vi "MoveAI.vi"(7 "ReturnHome(F)":bool, 8 "error in (no error)":errorcluster, 10 "Ball":refnum<class "PongBall.lvclass">, 11 "BouncePanel in":refnum<class "BouncePanel.lvclass">) -> (0 "error out":errorcluster, 3 "BouncePanel out":refnum<class "BouncePanel.lvclass">)   [LabVIEW 2019, in "RT_Game.lvlib" / "BouncePanel.lvclass"]
uses:
  BouncePanel.lvclass
  C:/Users/FreshBob/Dropbox/VIs/myRIO_GameConsole/RT/RT_Game/PongPanel/PongPanel.lvclass
  C:/Users/FreshBob/Dropbox/VIs/myRIO_GameConsole/RT/RT_Game/GameObject/GameObject.lvclass
  PongBall/PongBall.lvclass
  PongPanel/PongPanel.lvclass/PongPanel.ctl
  GameObject/GameObject.lvclass/GameObject.ctl
  PongPanel/Read StartPos.vi
  GameObject/Read Velocity.vi
  PongPanel/PongPanel.lvclass
  GameObject/GameObject.lvclass
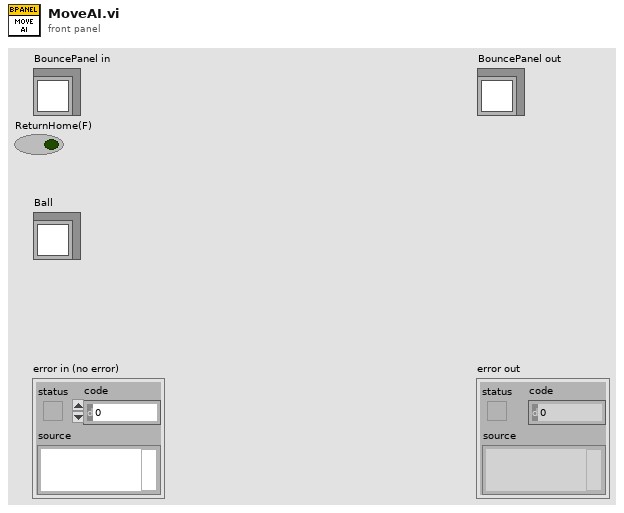
[diagram p1: front panel]
types:
  T1 = typedef "RT_Game.lvlib/Engine.lvclass/Coordinate.ctl" = cluster{"x":dbl, "y":dbl}
  T2 = typedef "Velocity.ctl" = cluster{"x":dbl, "y":dbl}
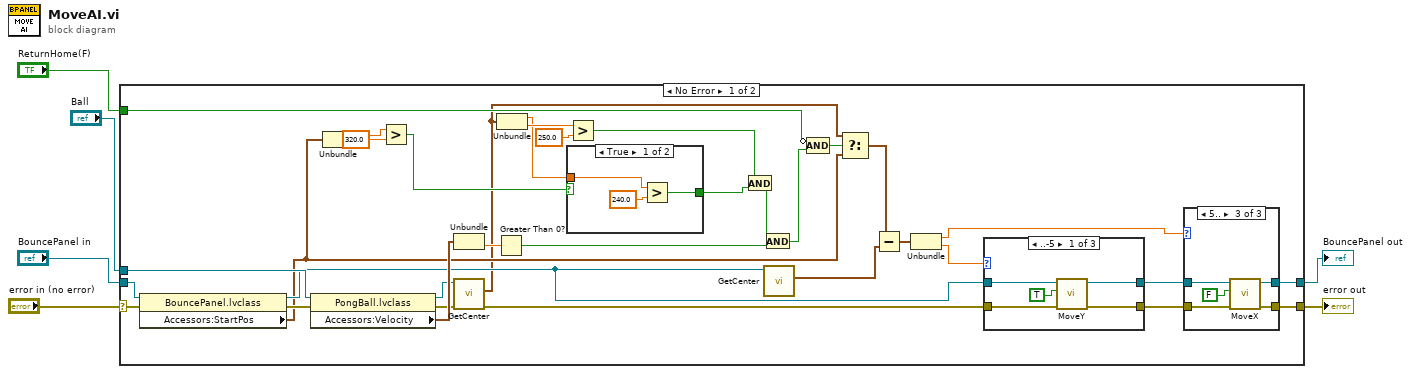
[diagram p0: block diagram]
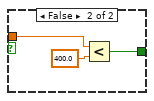
[diagram p2: hidden frame]
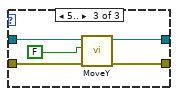
[diagram p4: hidden frame]
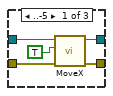
[diagram p5: hidden frame]
diagram:
  n1 = case shown="No Error" "error in (no error)" {
    selector: "error in (no error)" -> [w27 w72]
    tunnel: [w40 w72] -> w3
    tunnel: [w39 w71] -> w4
    tunnel: "BouncePanel in" -> [w22 w71]
    tunnel: "Ball" -> [w38 _]
    tunnel: "ReturnHome(F)" -> [w21 _]
    frame No Error {
      n2 = property class="BouncePanel.lvclass"(reference=w22, error in=w27) -> (reference out=w20:refnum<class "BouncePanel.lvclass">, error out=w23:errorcluster, "Accessors:StartPos"=w16:T1)
      n3 = property class="PongBall.lvclass"(reference=w38, error in=w23) -> (reference out=w35:refnum<class "PongBall.lvclass">, error out=w36:errorcluster, "Accessors:Velocity"=w37:T2)
      n4 = Unbundle(w16) -> ("x"=w15:dbl)  [unwired: 1 out]
      n5 = Greater?(x=w15, y=320.0) -> (0:w13:bool)
      n6 = Unbundle(w37) -> ("y"=w19:dbl)  [unwired: 1 out]
      n7 = call "GetCenter.vi"("error in (no error)"=w36, "GameObject in"=w35) -> ("error out"=w29:errorcluster, "center_pos"=w11:T1)  [unwired: 7 in, 1 out]
      n8 = Greater Than 0?(x=w19) -> (x > 0?=w26:bool)
      n9 = Unbundle(w11) -> ("x"=w12:dbl, "y"=w18:dbl)
      n10 = case shown="True" w13 {
        tunnel: w12 -> [w42 w45]
        tunnel: [w41 w44] -> w7
        frame True {
          n11 = Greater?(x=w42, y=240.0) -> (0:w41:bool)
        }
        frame False {
          n12 = Less?(x=w45, y=400.0) -> (x < y?=w44:bool)
        }
      }
      n13 = Greater?(x=w18, y=250.0) -> (0:w24:bool)
      n14 = And(x=w24, y=w7) -> (x .and. y?=w8:bool)
      n15 = And(x=w8, y=w26) -> (x .and. y?=w25:bool)
      n16 = call "GetCenter.vi"("GameObject in"=w20) -> ("center_pos"=w10:T1)  [unwired: 8 in, 2 out]
      n17 = Compound Arithmetic op=AND(invert w21, w25) -> (w28:bool)
      n18 = Select(t=w11, s=w28, f=w16) -> (s? t:f=w30:T1)
      n19 = Subtract(x=w30, y=w10) -> (x-y=w32:T1)
      n20 = Unbundle(w32) -> ("x"=w9:dbl, "y"=w31:dbl)
      n21 = case shown="..-5" w31 {
        tunnel: [w50 w52 w58] -> w34
        tunnel: [w48 w53 w57] -> w33
        tunnel: w29 -> [w51 w52 w56]
        tunnel: w20 -> [w49 w53 w55]
        frame ..-5 {
          n22 = call "MoveY.vi"("error in (no error)"=w51, "Up?"=TRUE, "PongPanel in"=w49) -> ("error out"=w50:errorcluster, "PongPanel out"=w48:refnum<class "BouncePanel.lvclass">)  [unwired: 7 in]
        }
        frame 0, Default {
        }
        frame 5.. {
          n23 = call "MoveY.vi"("error in (no error)"=w56, "Up?"=FALSE, "PongPanel in"=w55) -> ("error out"=w58:errorcluster, "PongPanel out"=w57:refnum<class "BouncePanel.lvclass">)  [unwired: 7 in]
        }
      }
      n24 = case shown="5.." w9 {
        tunnel: w34 -> [w63 w64 w70]
        tunnel: [w62 w64 w69] -> w40
        tunnel: w33 -> [w61 w65 w68]
        tunnel: [w60 w65 w67] -> w39
        frame ..-5 {
          n25 = call "MoveX.vi"("error in (no error)"=w63, "Left?"=TRUE, "PongPanel in"=w61) -> ("error out"=w62:errorcluster, "PongPanel out"=w60:refnum<class "BouncePanel.lvclass">)  [unwired: 7 in]
        }
        frame 0, Default {
        }
        frame 5.. {
          n26 = call "MoveX.vi"("error in (no error)"=w70, "Left?"=FALSE ("Up?"), "PongPanel in"=w68) -> ("error out"=w69:errorcluster, "PongPanel out"=w67:refnum<class "BouncePanel.lvclass">)  [unwired: 7 in]
        }
      }
    }
    frame Error {
    }
  }
  "error out" <- w3
  "BouncePanel out" <- w4
